vi "Generate.vi"(8 "error in (no error)":errorcluster, 11 "Composite Waveform in":refnum<class "Composite Waveform.lvclass">) -> (0 "error out":errorcluster, 3 "Composite Waveform out":refnum<class "Composite Waveform.lvclass">)   [LabVIEW 2020, in "Composite Waveform.lvclass"]
uses:
  Composite Waveform.lvclass
  Composite Waveform.lvclass/Composite Waveform.ctl
  Analog Waveform/Analog Waveform.lvclass
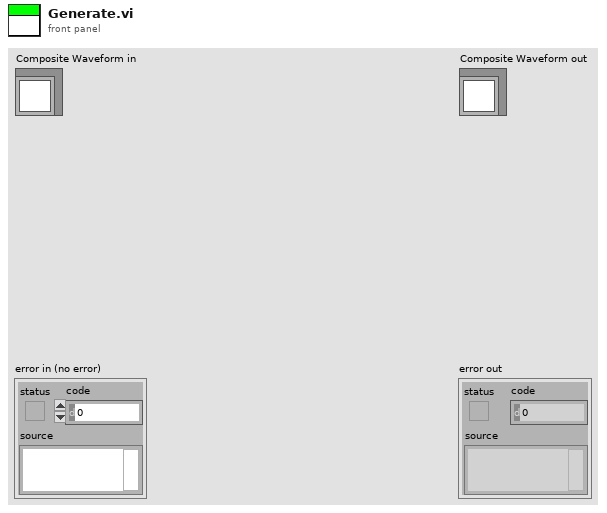
[diagram p1: front panel]
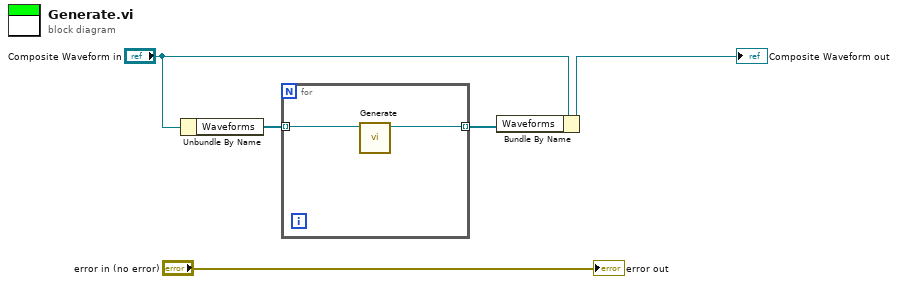
[diagram p0: block diagram]
diagram:
  n1 = Unbundle By Name("Composite Waveform in") -> ("Waveforms"=w3:refnum<class "Analog Waveform.lvclass">[])
  n2 = for {
    tunnel: w3 -> [w7] mode=indexing
    tunnel: [w6] -> w1 mode=indexing
    n3 = call-dynamic "Generate.vi"("Analog Waveform in"=w7) -> ("Analog Waveform out"=w6:refnum<class "Analog Waveform.lvclass">)  [unwired: 9 in, 1 out]
  }
  n4 = Bundle By Name(cluster="Composite Waveform in", "Waveforms"=w1) -> (→"Composite Waveform out":refnum<class "Composite Waveform.lvclass">)
  "error out" <- "error in (no error)"
